vi "Process.vi"(8 "error in":errorcluster, 11 "Instrument.Lockin":refnum<class "Instrument.Lockin.lvclass">) -> (0 "error out":errorcluster, 3 "Instrument.Lockin out":refnum<class "Instrument.Lockin.lvclass">)   [LabVIEW 2019, in "Instrument.Lockin.lvlib" / "Instrument.Lockin.lvclass"]
doc: "---------------------------------------------------------------\nJKI State Machine Objects™\nhttp://jki.net/state-machine-objects/\nCopyright (C) 2005-2015, JKI <info@jki.net>\nALL RIGHTS RESERVED"
uses:
  Instrument.Lockin.lvclass
  C:/Program Files/National Instruments/LabVIEW 2019/vi.lib/JKI/JKI SMO/SMO/SMO.lvclass
  C:/Program Files/National Instruments/LabVIEW 2019/user.lib/LevyLab/Instrument Framework/Instrument/Instrument.lvclass
  Typedefs/API/Lockin.Commands.Local--Enum.ctl
  Instrument.Lockin.lvclass/Instrument.Lockin.ctl
  Typedefs/Lockin.Logging Mode--Enum.ctl
  Instrument.DAQ/Typedefs/PublicEvents--DAQ.getSweepWaveforms.ctl
  <vilib>/JKI/JKI SMO/SMO/SMO.lvclass/SMO.ctl
  Instrument.DAQ/Typedefs/Get State-enum.ctl
  26abb908-d0dd-4bb2-b0ae-9417a76ac08a.vi
  58bdca10-aee7-4643-9696-ab134e43fedf.vi
  57cf7fb7-944b-4fe2-b1a2-0684563889c1.vi
  f640c324-6c77-497d-a9f4-fdf294fa3808.vi
  2ccda5d8-d2df-4877-8897-cb36dbf858a1.vi
  7ebf71aa-15a6-4da8-8ab8-2681a3011f9e.vi
  befd05cc-8908-477d-a2f5-b8fbe5183ab0.vi
  4dcf9d6e-caf6-43ae-ab2a-813b64901b82.vi
  0479806f-3f82-4f4d-965e-31251a6a8c57.vi
  26abb908-d0dd-4bb2-b0ae-9417a76ac08a.vi/90a97669-4453-472b-bdf1-7bcd8eb08246.vi
  26abb908-d0dd-4bb2-b0ae-9417a76ac08a.vi/b26fcf18-2a8e-4202-9f3a-794c759f590f.vi
  58bdca10-aee7-4643-9696-ab134e43fedf.vi/a5cadab5-4a81-4843-8cd1-df529f160719.vi
  58bdca10-aee7-4643-9696-ab134e43fedf.vi/d6a5cc56-11f2-457d-8496-f6582433bdb5.vi
  57cf7fb7-944b-4fe2-b1a2-0684563889c1.vi/c78e9024-35b9-404a-847a-34b4f0e1b7cd.vi
  57cf7fb7-944b-4fe2-b1a2-0684563889c1.vi/9cccbff1-3b31-4ba5-974e-4119a5b66697.vi
  f640c324-6c77-497d-a9f4-fdf294fa3808.vi/fd9c0a75-bb1c-4df5-b428-97473e186f85.vi
  f640c324-6c77-497d-a9f4-fdf294fa3808.vi/5a332ac2-f3ee-43b7-a900-88e315d2e26c.vi
  2ccda5d8-d2df-4877-8897-cb36dbf858a1.vi/5836e187-7c61-41ed-8ee9-21d612ef42f8.vi
  2ccda5d8-d2df-4877-8897-cb36dbf858a1.vi/e16ae26d-577b-44d4-8830-38d114a60ef0.vi
  7ebf71aa-15a6-4da8-8ab8-2681a3011f9e.vi/4fe2dc9d-9353-45a3-b3dd-066009c5f601.vi
  7ebf71aa-15a6-4da8-8ab8-2681a3011f9e.vi/a83d1b05-35e4-4348-922d-f6ae74c7e255.vi
  befd05cc-8908-477d-a2f5-b8fbe5183ab0.vi/289e6158-3360-40af-af80-2e4dcd9b67a9.vi
  befd05cc-8908-477d-a2f5-b8fbe5183ab0.vi/5139ce6f-e826-4046-ae95-8880b2f2c8e2.vi
  4dcf9d6e-caf6-43ae-ab2a-813b64901b82.vi/c32a3efa-f786-486f-88c4-db6f71449899.vi
  4dcf9d6e-caf6-43ae-ab2a-813b64901b82.vi/a7bed843-5626-489a-9ac6-3c2874ac1268.vi
  0479806f-3f82-4f4d-965e-31251a6a8c57.vi/c63cbaba-d6ce-4e6f-84ba-6c88dbec8892.vi
  0479806f-3f82-4f4d-965e-31251a6a8c57.vi/12d99530-24f6-4df4-a18b-ab3b3e1e63e9.vi
  <vilib>/JKI/JKI SMO/SMO/Private/ReftoDVR--SMO.vi
  <vilib>/Utility/Data Type/Get Type Information.vi
  <vilib>/Utility/Data Type/Get Numeric Information.vi
  <userlib>/_OpenG.lib/lvdata/lvdata.llb/Unwrap VVariant__ogtk.vi
  <vilib>/JDP Science/JSONtext/Variant to JSON Text.vi
  <userlib>/LevyLab/Instrument Framework/Instrument/API/Instrument.sendMessageToProcess (string).vi
  <vilib>/JDP Science/JSONtext/LVClass Serializer/JSONtext LVClass Serializer.lvclass
  <userlib>/LevyLab/Instrument Framework/Instrument Types/Lockin/Instrument.LockinAPI.lvclass
  <userlib>/LevyLab/Debug/Debug.lvlib
  <userlib>/LevyLab/Instrument Framework/Instrument/Instrument.lvclass
  Instrument.DAQ/Instrument.DAQ.lvclass
  <vilib>/JKI/JKI SMO/SMO/SMO.lvclass
panel:
  in  "LOG":bool
  out "String":string
  # "Multichannel Lockin"
  # "For instructions on how to use the JKI State Machine Objects, examples and video tutorials, visit:\nhttp://jki.net/state-machine-objects/\n\nJKI State Machine Objects™\nhttp://jki.net/state-machine-objects/\nCopyright (C) 2005-2015, JKI <info@jki.net>\nALL RIGHTS RESERVED"
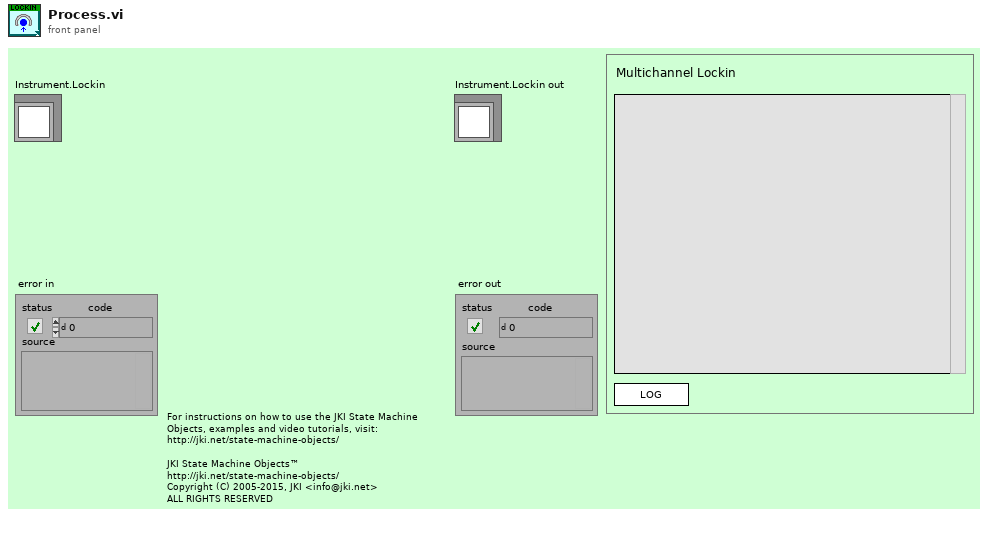
[diagram p1: front panel]
types:
  T1 = typedef "Instrument.Lockin.lvlib/Instrument.Lockin.lvclass/Lockin.Commands.Local--Enum.ctl" = enum16{"autoConfigureDAQ", "setSimulationMode", "zeroPhase", "setCalibration", "setPreFilter", "setLinkFrequencies", "setLimitAmplitude", "setLimitDC", "setSamplingDecimationPreDSP", "setSamplingDecimationPostDSP", "setSamplingMode", "setSamplingFsMultiplier", "setSamplingFsOutput", "setSamplingRefreshRate", "setData_State", "setData_DAQ", "setData_Sampling", "setData_Waveforms", "setData_Results", "setData_SweepWaveforms", "setData_AIChannels", "setData_AOChannels", "setData_REFChannels", "setData_InputGain", "setData_OutputGain", "showUI", "setAI", "setOffset", "setOffsetMode"}
  T2 = typedef "Instrument.Lockin.lvlib/Instrument.Lockin.lvclass/Lockin.Logging Mode--Enum.ctl" = enum16{"enabled", "disabled"}
  T3 = enum32{"invalid app kind", "Development System", "Run Time System", "Student Edition", "Embedded LabVIEW", "Evaluation", "Custom"}
  T4 = enum32{"Invalid", "Standard", "Closed", "Hidden", "Minimized", "Maximized"}
  T5 = typedef "Instrument.Lockin.lvlib/Instrument.DAQ.lvclass/Get State-enum.ctl" = enum16{"idle", "created", "started", "stopped", "sweeping"}
  T6 = typedef "Instrument.Lockin.lvlib/Instrument.DAQ.lvclass/PublicEvents--DAQ.getSweepWaveforms.ctl" = cluster{"AO_wfm":waveform(dbl)[], "AI_wfm":waveform(dbl)[], "X_wfm":waveform(dbl)[], "Y_wfm":waveform(dbl)[]}
  T7 = typedef "SMO.lvclass/SMOState --Enum.ctl" = enum16{"unknown", "Created", "Started", "Stopped"}
  T8 = cluster{"Core":cluster{"Current VI Reference":refnum<vi>, "Close Panel on Exit?":bool, "Last Error":cluster{"error":errorcluster, "previous state":string, "remaining states":string}, "Shutdown?":bool}, "SelfRef":refnum<class "Instrument.Lockin.lvclass">, "SweepWaveformsBuffer":T6}
  T9 = typedef "Instrument.Lockin.lvlib/Instrument.DAQ.lvclass/DAQ.Configuration--Cluster--Array.ctl" = T10[]
  T10 = typedef "Instrument.Lockin.lvlib/Instrument.DAQ.lvclass/DAQ.Configuration--Cluster.ctl" = cluster{"Device":string, "AO.Ch":string, "AO.Range":T11, "AI.Ch":string, "AI.Range":T12, "AI.Coupling":T13}
  T11 = typedef "Instrument.Lockin.lvlib/Instrument.DAQ.lvclass/DAQ.Config.AO.Range--enum.ctl" = enum16{"±0.1", "±1.0", "±10.0"}
  T12 = typedef "Instrument.Lockin.lvlib/Instrument.DAQ.lvclass/DAQ.Config.AI.Range--enum.ctl" = enum16{"±0.316", "±1.00", "±3.16", "±10.0", "±31.6", "±42.4"}
  T13 = typedef "Instrument.Lockin.lvlib/Instrument.DAQ.lvclass/DAQ.Config.AI.Coupling--enum.ctl" = u16
  T14 = typedef "Instrument.Lockin.lvlib/Instrument.DAQ.lvclass/DAQ.Config.AO--Cluster--Array.ctl" = T15[]
  T15 = typedef "Instrument.Lockin.lvlib/Instrument.DAQ.lvclass/DAQ.Config.AO--Cluster.ctl" = cluster{"Channels":tag, "Range":T11, "output terminal configuration":i32, "Type":T16}
  T16 = typedef "Instrument.Lockin.lvlib/Instrument.DAQ.lvclass/DAQ.Type--enum.ctl" = enum16{"None", "USB-4431", "PXI-446x"}
  T17 = typedef "Instrument.Lockin.lvlib/Instrument.DAQ.lvclass/DAQ.Config.AI--Cluster--Array.ctl" = T18[]
  T18 = typedef "Instrument.Lockin.lvlib/Instrument.DAQ.lvclass/DAQ.Config.AI--Cluster.ctl" = cluster{"Channels":tag, "Coupling":T13, "Range":T12, "input terminal configuration":i32, "Type":T16}
  T19 = typedef "Instrument.Lockin.lvlib/Instrument.DAQ.lvclass/DAQ.Sampling--Cluster.ctl" = cluster{"Sampling":T20, "sample mode":i32, "Fs Mode":T21, "Fs Multiplier":dbl, "Refresh Rate (Hz)":dbl, "Decimation.PreDSP":i32, "Decimation.PostDSP":i32, "Fs.Output":dbl}
  T20 = typedef "Instrument.Lockin.lvlib/Instrument.DAQ.lvclass/DAQ.Sampling.Sampling--Cluster.ctl" = cluster{"Fs":dbl, "#s":i32}
  T21 = typedef "Instrument.Lockin.lvlib/Instrument.DAQ.lvclass/DAQ.Sampling.Fs Mode--enum.ctl" = enum16{"Manual", "Auto Fs", "Max Fs"}
  T22 = typedef "Instrument.Lockin.lvlib/Instrument.DAQ.lvclass/AI.Channel--Cluster--Array.ctl" = T23[]
  T23 = typedef "Instrument.Lockin.lvlib/Instrument.DAQ.lvclass/AI.Channel--Cluster.ctl" = cluster{"Enable?":bool, "Channel":i32, "References":i32[]}
  T24 = typedef "Instrument.Lockin.lvlib/Instrument.DAQ.lvclass/AO.Channel--Cluster--Array.ctl" = T25[]
  T25 = typedef "Instrument.Lockin.lvlib/Instrument.DAQ.lvclass/AO.Channel--Cluster.ctl" = cluster{"Enable?":bool, "Channel":i32, "Amplitude":dbl, "Offset":dbl, "Frequency":dbl, "Phase":dbl, "Function":T26, "Sweeping?":bool}
  T26 = typedef "Instrument.Lockin.lvlib/Instrument.DAQ.lvclass/AO.Channel.Function--Enum.ctl" = enum16{"Sine", "Triangle", "Square"}
  T27 = typedef "Instrument.Lockin.lvlib/Instrument.DAQ.lvclass/REF.Channel--Cluster--Array.ctl" = T28[]
  T28 = typedef "Instrument.Lockin.lvlib/Instrument.DAQ.lvclass/REF.Channel--Cluster.ctl" = cluster{"Enable?":bool, "Channel":i32, "Frequency":dbl, "Phase":dbl, "TC":dbl, "Roll-Off":i32}
  T29 = typedef "Instrument.Lockin.lvlib/Instrument.DAQ.lvclass/PublicEvents--DAQ.getWaveforms.ctl" = cluster{"AO_wfm":waveform(dbl)[], "AI_wfm":waveform(dbl)[], "Ref_X_wfm":waveform(dbl)[], "Ref_Y_wfm":waveform(dbl)[], "X_wfm":waveform(dbl)[], "Y_wfm":waveform(dbl)[]}
  T30 = typedef "Instrument.Lockin.lvlib/Instrument.DAQ.lvclass/Results--Cluster.ctl" = cluster{"Time Stamp":timestamp, "Results (Dictionary)":cluster{"key":string, "value":dbl}[]}
  T31 = typedef "Instrument.Lockin.lvlib/Instrument.DAQ.lvclass/DeviceInfo--Cluster.ctl" = cluster{"DeviceName":string, "DevIsSimulated":bool, "DeviceSerialNumber":u32, "ProductType":string, "ProductCategory":i32, "ProductNumber":u32, "ChassisNumber":u32, "SlotNumber":u32, "ChassisName":string, "ChassisSerialNumber":u32}
  T32 = cluster{"Current VI Reference":refnum<vi>, "Close Panel on Exit?":bool, "Last Error":cluster{"error":errorcluster, "previous state":string, "remaining states":string}, "Shutdown?":bool}
  T33 = typedef "Debug.lvlib/Attribute.Debug.lvclass/DebugBehavior.ctl" = enum16{"Normal", "Debug"}
  T34 = typedef "SMO.lvclass/Protected Events.ctl" = cluster{"StopProcesses":refnum<user-event>, "AbortProcesses":refnum<user-event>, "Config Changed":refnum<user-event>, "Dependency":refnum<user-event>}
  T35 = typedef "SMO.lvclass/Public Events.ctl" = cluster{"Error":refnum<user-event>, "State":refnum<user-event>, "Reserve State":refnum<user-event>}
  T36 = typedef "Instrument.Lockin.lvlib/Instrument.DAQ.lvclass/PublicEvents--Cluster.ctl" = cluster{"getAIChannels":refnum<user-event>, "getAOChannels":refnum<user-event>, "getREFChannels":refnum<user-event>, "getWaveforms":refnum<user-event>, "getResults":refnum<user-event>, "getSweepWaveforms":refnum<user-event>, "getCalibration":refnum<user-event>, "getDAQState":refnum<user-event>, "getDAQconfig":refnum<user-event>, "getInputGain":refnum<user-event>, "getOutputGain":refnum<user-event>, "getInputOffset":refnum<user-event>, "getSampling":refnum<user-event>, "getSweepChannels":refnum<user-event>, "getDeviceIDN":refnum<user-event>}
  T37 = typedef "Instrument.Lockin.lvlib/Instrument.Lockin.lvclass/PrivateEvents--Cluster.ctl" = cluster{"Logging":refnum<user-event>}
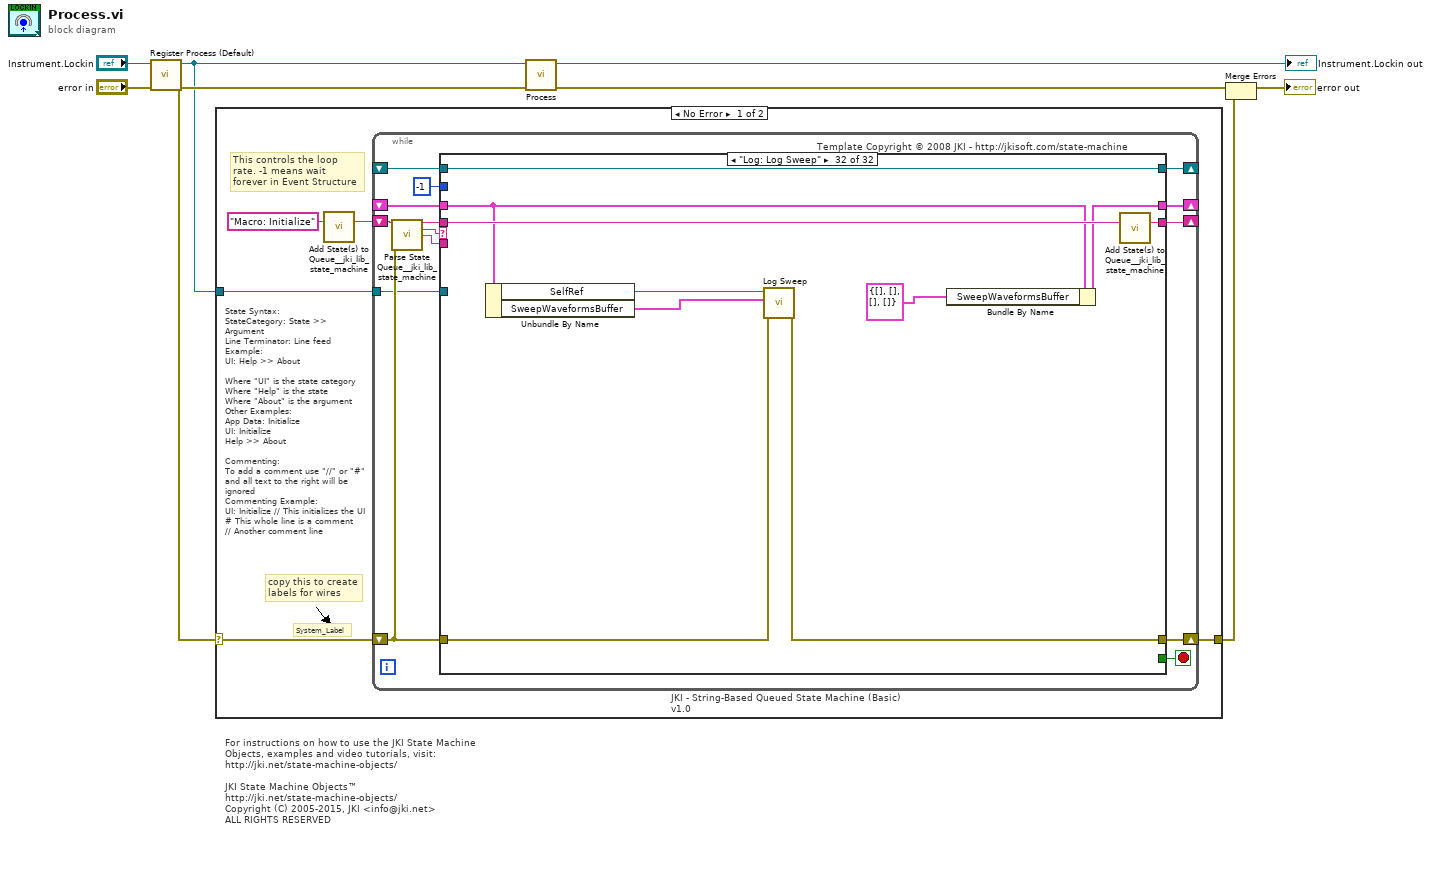
[diagram p0: block diagram]
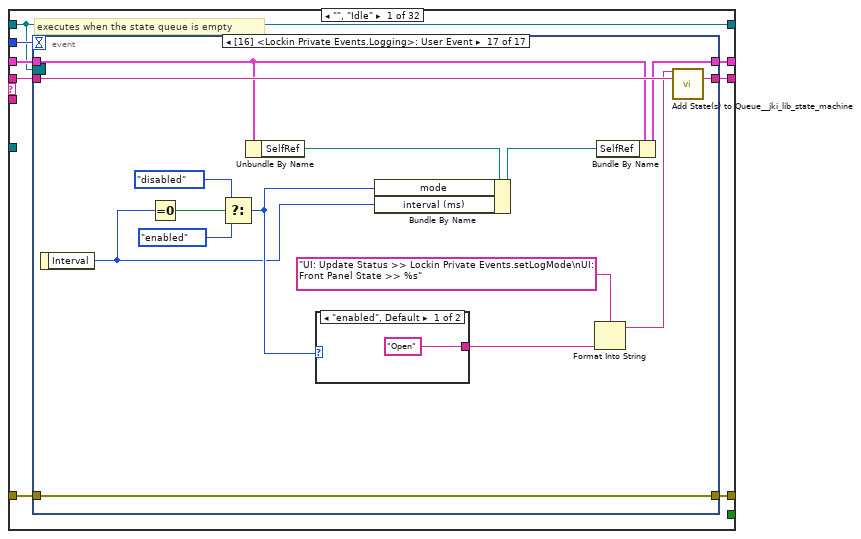
[diagram p2: hidden frame]
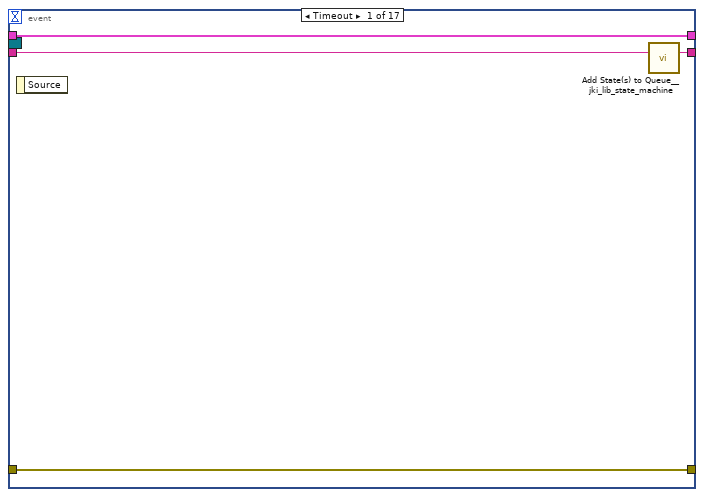
[diagram p3: hidden frame]
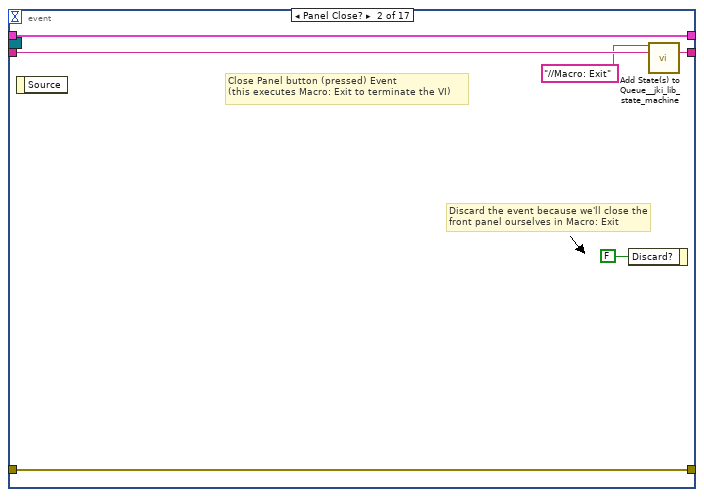
[diagram p4: hidden frame]
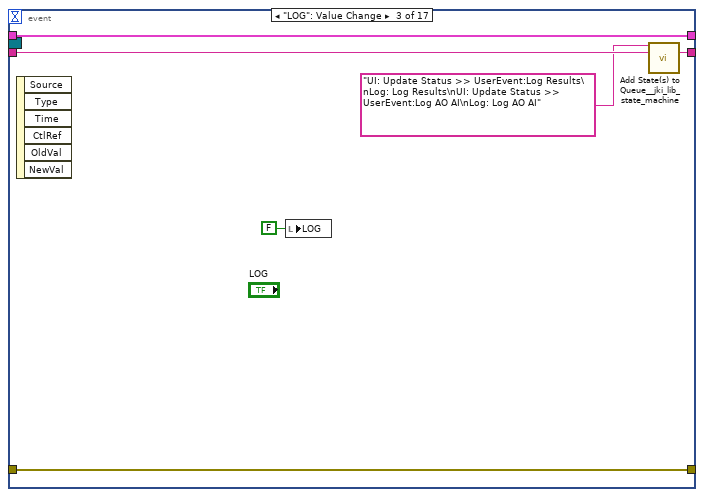
[diagram p5: hidden frame]
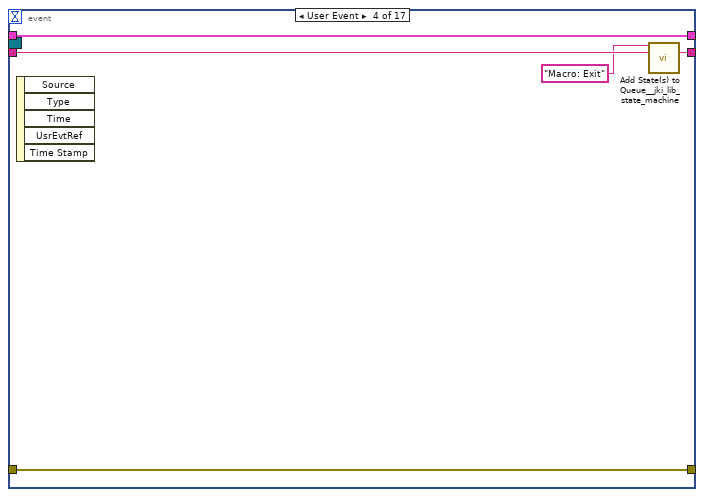
[diagram p6: hidden frame]
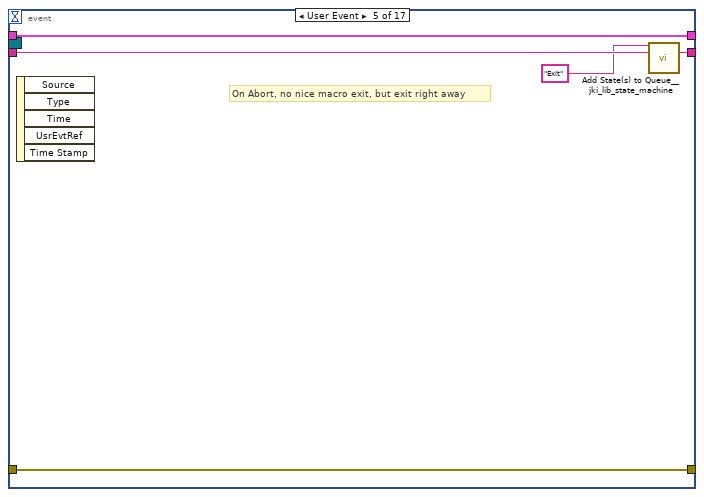
[diagram p7: hidden frame]
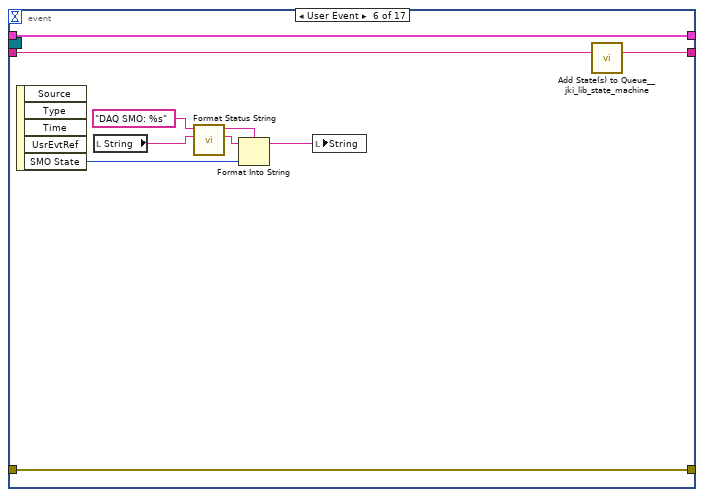
[diagram p8: hidden frame]
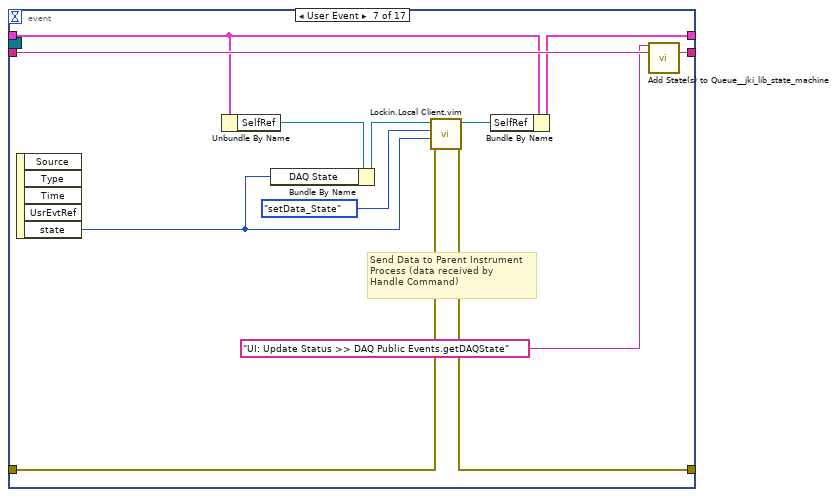
[diagram p9: hidden frame]
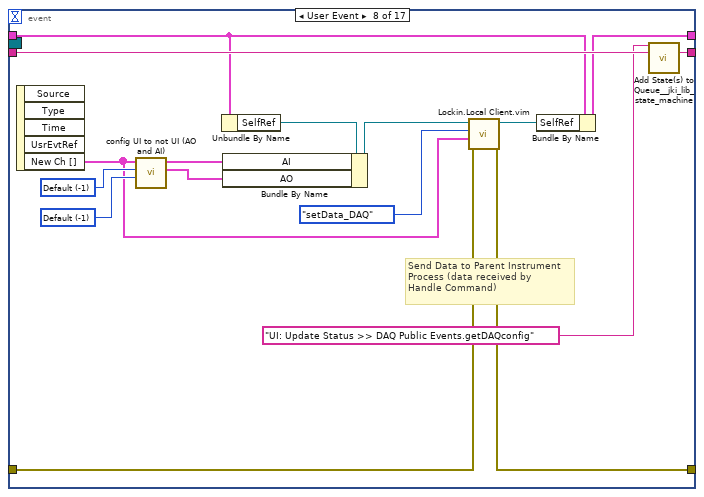
[diagram p10: hidden frame]
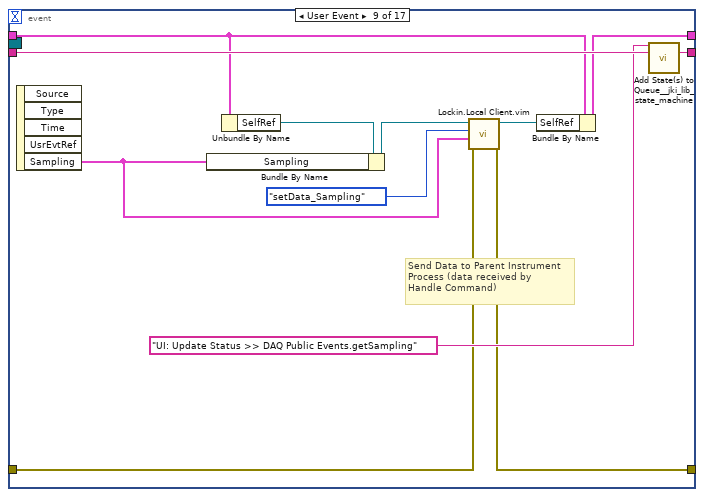
[diagram p11: hidden frame]
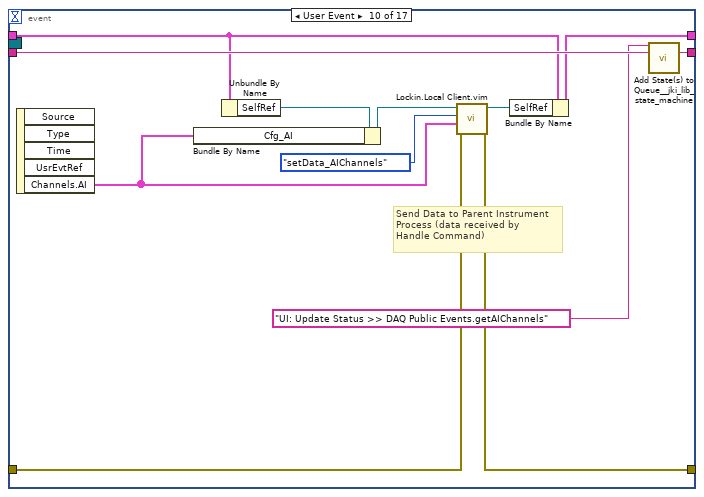
[diagram p12: hidden frame]
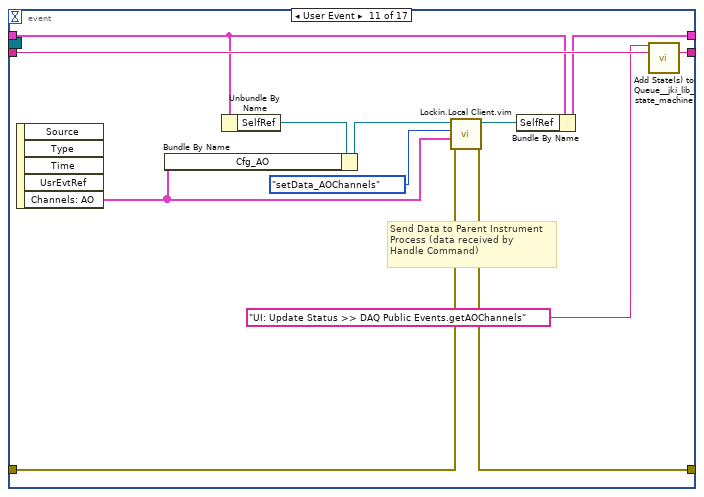
[diagram p13: hidden frame]
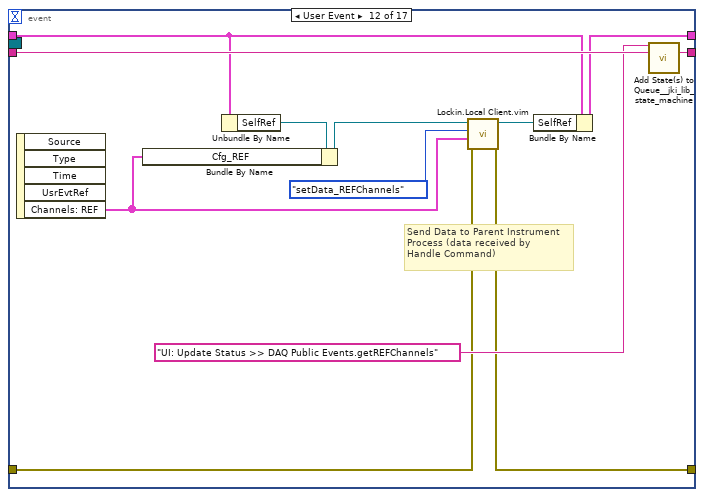
[diagram p14: hidden frame]
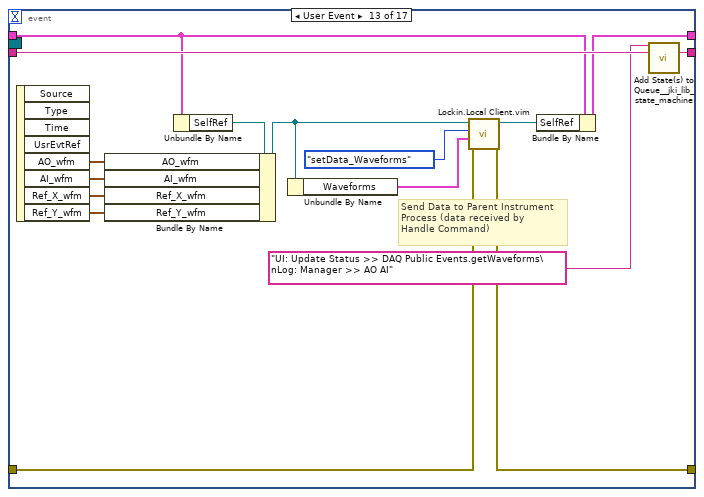
[diagram p15: hidden frame]
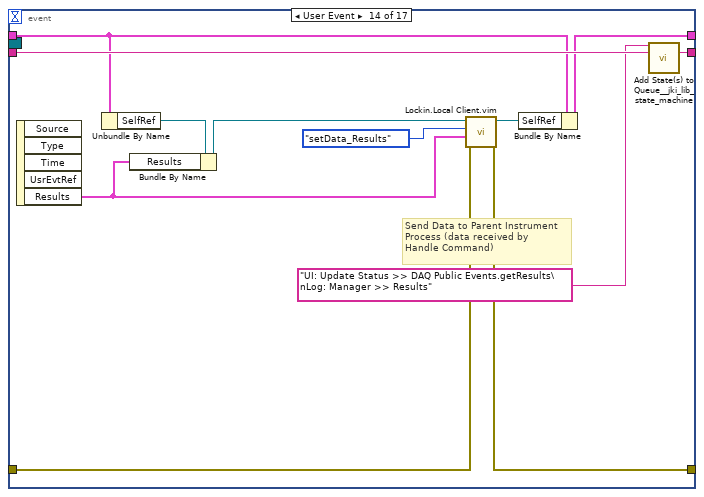
[diagram p16: hidden frame]
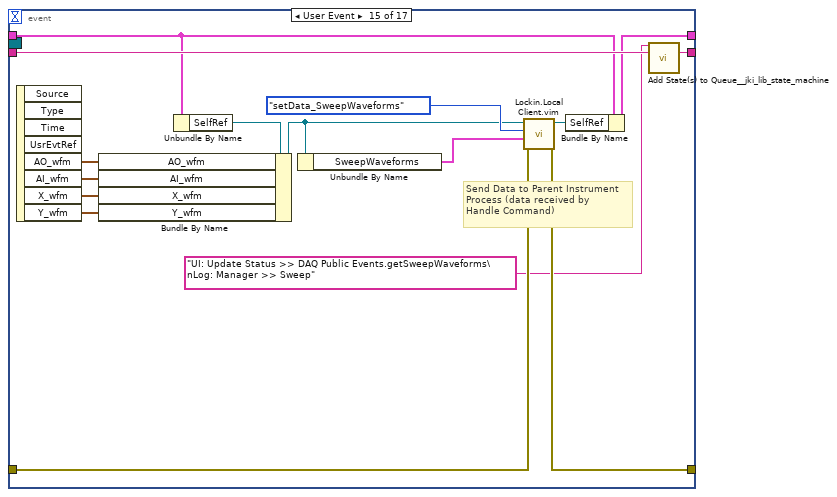
[diagram p17: hidden frame]
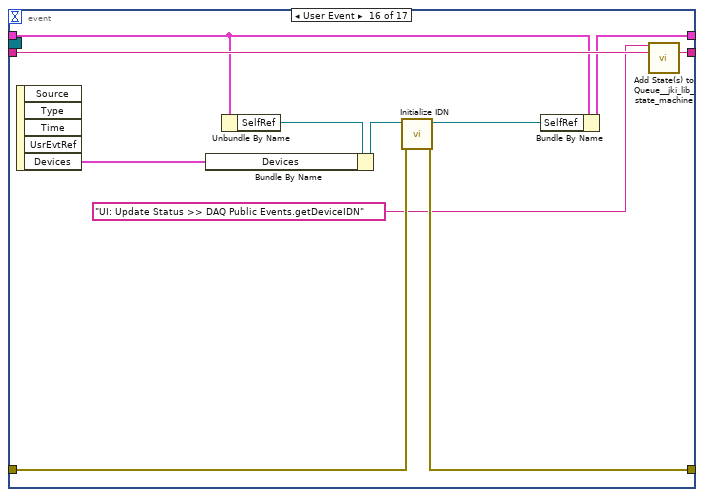
[diagram p18: hidden frame]
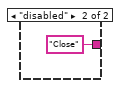
[diagram p19: hidden frame]
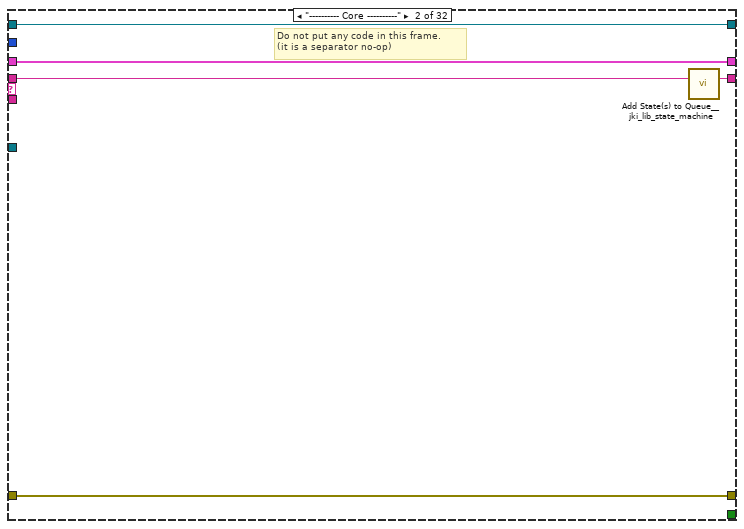
[diagram p20: hidden frame]
diagram:
  # "For instructions on how to use the JKI State Machine Objects, examples and video tutorials, visit:\nhttp://jki.net/state-machine-objects/\n\nJKI State Machine Objects™\nhttp://jki.net/state-machine-objects/\nCopyright (C) 2005-2015, JKI <info@jki.net>\nALL RIGHTS RESERVED"
  n1 = call <vilib>:"Register Process (Default).vi"("error in (no error)"="error in", "SMO"="Instrument.Lockin") -> ("error out"=w5:errorcluster, "SelfRef"=w4:refnum<class "Instrument.Lockin.lvclass">)  [unwired: 8 in]
  n2 = case shown="No Error" w5 {
    selector: w5 -> [w10 w574]
    tunnel: w4 -> [w11 _]
    tunnel: [w9 w574] -> w1
    frame No Error {
      # "State Syntax:\nStateCategory: State >> Argument\nLine Terminator: Line feed\nExample:\nUI: Help >> About\n\nWhere \"UI\" is the state category\nWhere \"Help\" is the state\nWhere \"About\" is the argument\nOther Examples:\nApp Data: Initialize\nUI: Initialize\nHelp >> About\n\nCommenting:\nTo add a comment use \"//\" or \"#\" and all text to the right will be ignored\nCommenting Example:\nUI: Initialize // This initializes the UI\n# This whole line is a comment\n// Another comment line"
      # "copy this to create labels for wires"
      # "This controls the loop rate. -1 means wait forever in Event Structure"
      # "System_Label"
      n3 = call <vilib>:"Add State(s) to Queue__jki_lib_state_machine.vi"("State(s) in (\"\")"="Macro: Initialize") -> ("States Out"=w13:string)  [unwired: 14 in]
      n4 = while "JKI - String-Based Queued State Machine (Basic) v1.0" {
        shift-right: [w20] -> _
        shift-left: _ -> [w19]
        shift-right: [w23] -> w9
        shift-left: w10 -> [w17]
        shift-right: [w22] -> _
        shift-left: w13 -> [w24]
        tunnel: w11 -> [w16]
        shift-right: [w15] -> _
        shift-left: _ -> [w14]
        stop <- w21 stop-if-true
        # "Template Copyright © 2008 JKI - http://jkisoft.com/state-machine"
        n5 = call <vilib>:"Parse State Queue__jki_lib_state_machine.vi"("State Queue"=w24, "Error In (no error)"=w17) -> ("Remaining States"=w26:string, "Current State"=w27:string, "Arguments"=w25:string)  [unwired: 11 in]
        n6 = case shown="\"Log: Log Sweep\"" w27 {
          selector: w27 -> [_ _ w226 _ _ _ _ _ _ _ _ _ _ _ _ _ _ _ _ _ _ _ _ _ _ _ _ _ _ _ _ _]
          tunnel: w26 -> [w35 w224 w230 w249 w251 w268 w273 w284 w291 w311 w316 w324 w331 w340 w347 w363 w395 w404 w416 w435 w456 w461 w472 w477 w494 w500 w505 w516 w549 w556 w563 w573]
          tunnel: w25 -> [_ _ _ _ _ _ _ _ _ _ _ _ w325 w332 w341 w357 _ _ _ _ _ _ _ _ _ _ _ w506 _ _ _ _]
          tunnel: w19 -> [w33 w221 w228 w240 w258 w264 w270 _ w286 w298 w313 w322 w328 w337 w345 w359 w392 w396 w405 w424 w441 w458 w469 w474 w488 w498 w501 w512 w546 w553 w560 w565]
          tunnel: [w32 w222 w232 w246 errorcluster {"status"=FALSE, "code"=0, "source"=""} ("No error") w263 w271 w280 w287 w309 w314 w319 w329 w338 w342 w360 w393 w398 w414 w422 w454 w459 w463 w475 w490 w496 w502 w513 w545 w552 w557 w568] -> w23
          tunnel: w17 -> [w31 w222 w231 w246 w260 _ w271 w280 w288 w309 w314 w318 w329 w338 w343 w361 w393 w398 w414 w421 w454 w459 w464 w475 w486 w496 w502 w513 w544 w550 w558 w569]
          tunnel: [w34 w223 w229 w248 w256 w267 w272 w283 w290 w310 w315 w323 w330 w339 w346 w362 w394 w403 w415 w434 w455 w460 w471 w476 w493 w499 w504 w515 w548 w555 w562 w572] -> w22
          tunnel: [_ _ _ _ _ TRUE _ _ _ _ _ _ _ _ _ _ _ _ _ _ _ _ _ _ _ _ _ _ _ _ _ _] -> w21
          tunnel: [w30 w221 w228 w247 w257 w264 w270 w282 w286 w299 w313 w322 w328 w337 w345 w359 w392 w396 w406 w425 w442 w458 w469 w474 w488 w498 w501 w512 w546 w553 w560 w566] -> w20
          tunnel: -1 ("Timeout") -> [w29 _ _ _ _ _ _ _ _ _ _ _ _ _ _ _ _ _ _ _ _ _ _ _ _ _ _ _ _ _ _ _]
          tunnel: w16 -> [_ _ _ _ _ _ _ w277 _ _ _ _ _ _ _ _ _ _ _ _ _ _ _ _ _ _ _ _ _ _ _ _]
          tunnel: [w28 w220 w225 w237 w262 w265 w269 w281 w285 w308 w312 w321 w327 w336 w344 w356 w391 w402 w413 w433 w448 w457 w470 w473 w492 w497 w503 w514 w547 w554 w561 w571] -> w15
          tunnel: w14 -> [w28 w220 w225 w237 w262 w265 w269 w281 w285 w308 w312 w321 w327 w336 w344 w356 w391 w402 w413 w433 w448 w457 w470 w473 _ w497 w503 w514 w547 w554 w561 w571]
          frame "", "Idle" {
            # "executes when the state queue is empty"
            n7 = event shown="[16] <Lockin Private Events.Logging>: User Event" {
              selector: w28 -> [_ _ _ _ _ _ _ _ _ _ _ _ _ _ _ _ _]
              dyn-events: _ -> [_ _ _ _ _ _ _ _ _ _ _ _ _ _ _ _ _]
              timeout: w29 -> [_ _ _ _ _ _ _ _ _ _ _ _ _ _ _ _ _]
              tunnel: w35 -> [w39 w45 w51 w56 w61 w69 w83 w99 w111 w123 w135 w147 w163 w175 w191 w202 w217]
              tunnel: [w38 w44 w50 w55 w60 w70 w82 w98 w110 w122 w134 w146 w162 w174 w190 w201 w216] -> w34
              tunnel: w33 -> [w36 w42 w48 w53 w58 w68 w80 w96 w108 w120 w132 w144 w160 w172 w188 w199 w214]
              tunnel: [w37 w43 w49 w54 w59 w67 w76 w86 w102 w117 w126 w137 w151 w170 w180 w194 w212] -> w32
              tunnel: w31 -> [w37 w43 w49 w54 w59 w67 w75 w85 w101 w116 w125 w136 w150 w169 w179 w193 w212]
              tunnel: [w36 w42 w48 w53 w58 w68 w81 w97 w109 w121 w133 w145 w161 w173 w189 w200 w215] -> w30
              event Timeout {
                n8 = event-data() -> ()  [unwired: 1 in, 1 out]
                n9 = call <vilib>:"Add State(s) to Queue__jki_lib_state_machine.vi"("State(s) in (\"\")"=w39) -> ("States Out"=w38:string)  [unwired: 14 in]
              }
              event Panel Close? {
                # "Discard the event because we'll close the front panel ourselves in Macro: Exit"
                # "Close Panel button (pressed) Event\n(this executes Macro: Exit to terminate the VI)"
                n10 = event-data() -> ()  [unwired: 1 in, 1 out]
                n11 = event-data("Discard?"=FALSE) -> ()  [unwired: 1 in, 1 out]
                n12 = call <vilib>:"Add State(s) to Queue__jki_lib_state_machine.vi"("State(s) in Front (\"\")"="//Macro: Exit", "State(s) in (\"\")"=w45) -> ("States Out"=w44:string)  [unwired: 13 in]
              }
              event "LOG": Value Change {
                n13 = event-data() -> ()  [unwired: 1 in, 6 out]
                n14 = local write "LOG"(FALSE ("LOG")) -> ()
                n15 = call <vilib>:"Add State(s) to Queue__jki_lib_state_machine.vi"("State(s) in Front (\"\")"="UI: Update Status >> UserEvent:Log Results\nLog: Log Results\nUI: Update Status >> UserEvent:Log AO AI\nLog: Log AO AI", "State(s) in (\"\")"=w51) -> ("States Out"=w50:string)  [unwired: 13 in]
              }
              event User Event {
                n16 = event-data() -> ()  [unwired: 1 in, 5 out]
                n17 = call <vilib>:"Add State(s) to Queue__jki_lib_state_machine.vi"("State(s) in Front (\"\")"="Macro: Exit", "State(s) in (\"\")"=w56) -> ("States Out"=w55:string)  [unwired: 13 in]
              }
              event User Event {
                # "On Abort, no nice macro exit, but exit right away"
                n18 = event-data() -> ()  [unwired: 1 in, 5 out]
                n19 = call <vilib>:"Add State(s) to Queue__jki_lib_state_machine.vi"("State(s) in Front (\"\")"="Exit", "State(s) in (\"\")"=w61) -> ("States Out"=w60:string)  [unwired: 13 in]
              }
              event User Event {
                n20 = event-data() -> ("SMO State"=w71:T7)  [unwired: 1 in, 4 out]
                n21 = local read "String"() -> (w64:string)
                n22 = call "Format Status String.vi"("initial string"=w64, "format string"="DAQ SMO: %s") -> ("initial string out"=w63:string, "format string out"=w62:string)  [unwired: 8 in]
                n23 = Format Into String(format string=w62, initial string=w63, w71) -> (resulting string=w66:string)  [unwired: 1 in, 1 out]
                n24 = local write "String"(w66) -> ()
                n25 = call <vilib>:"Add State(s) to Queue__jki_lib_state_machine.vi"("State(s) in (\"\")"=w69) -> ("States Out"=w70:string)  [unwired: 14 in]
              }
              event User Event {
                # "Send Data to Parent Instrument\nProcess (data received by\nHandle Command)"
                n26 = event-data() -> ("state"=w74:T5)  [unwired: 1 in, 4 out]
                n27 = Unbundle By Name(w80) -> ("SelfRef"=w73:refnum<class "Instrument.Lockin.lvclass">)
                n28 = Bundle By Name(cluster=w73, "DAQ State"=w74) -> (w72:refnum<class "Instrument.Lockin.lvclass">)
                n29 = call "Lockin.Local Client.vim"("error in (no error)"=w75, "Data"=w74, "Command"=Lockin.Commands.Local--Enum."setData_State" ("Enum"), "Instrument.Lockin in"=w72) -> ("error out"=w76:errorcluster, "Instrument.Lockin out"=w77:refnum<class "Instrument.Lockin.lvclass">)  [unwired: 6 in]
                n30 = Bundle By Name(cluster=w80, "SelfRef"=w77) -> (w81:T8)
                n31 = call <vilib>:"Add State(s) to Queue__jki_lib_state_machine.vi"("State(s) in Front (\"\")"="UI: Update Status >> DAQ Public Events.getDAQState" ("State(s) in Front (\"\")"), "State(s) in (\"\")"=w83) -> ("States Out"=w82:string)  [unwired: 13 in]
              }
              event User Event {
                w92 = -1 items=["Default"=-1, "RSE"=10083, "Differential"=10106, "Pseudodifferential"=12529] ("output terminal configuration")
                w93 = -1 items=["Default"=-1, "RSE"=10083, "NRSE"=10078, "Differential"=10106, "Pseudodifferential"=12529] ("input terminal configuration")
                # "Send Data to Parent Instrument\nProcess (data received by\nHandle Command)"
                n32 = event-data() -> ("New Ch []"=w87:T9)  [unwired: 1 in, 4 out]
                n33 = call "config UI to not UI (AO and AI).vi"("output terminal configuration"=w92, "input terminal configuration"=w93, "New Ch []"=w87) -> ("AO Config"=w90:T14, "AI Config"=w91:T17)  [unwired: 7 in]
                n34 = Unbundle By Name(w96) -> ("SelfRef"=w95:refnum<class "Instrument.Lockin.lvclass">)
                n35 = Bundle By Name(cluster=w95, "AI"=w91, "AO"=w90) -> (w89:refnum<class "Instrument.Lockin.lvclass">)
                n36 = call "Lockin.Local Client.vim"("error in (no error)"=w85, "Data"=w87, "Command"=Lockin.Commands.Local--Enum."setData_DAQ" ("Enum"), "Instrument.Lockin in"=w89) -> ("error out"=w86:errorcluster, "Instrument.Lockin out"=w88:refnum<class "Instrument.Lockin.lvclass">)  [unwired: 6 in]
                n37 = Bundle By Name(cluster=w96, "SelfRef"=w88) -> (w97:T8)
                n38 = call <vilib>:"Add State(s) to Queue__jki_lib_state_machine.vi"("State(s) in Front (\"\")"="UI: Update Status >> DAQ Public Events.getDAQconfig" ("State(s) in Front (\"\")"), "State(s) in (\"\")"=w99) -> ("States Out"=w98:string)  [unwired: 13 in]
              }
              event User Event {
                # "Send Data to Parent Instrument\nProcess (data received by\nHandle Command)"
                n39 = event-data() -> ("Sampling"=w100:T19)  [unwired: 1 in, 4 out]
                n40 = Unbundle By Name(w108) -> ("SelfRef"=w107:refnum<class "Instrument.Lockin.lvclass">)
                n41 = Bundle By Name(cluster=w107, "Sampling"=w100) -> (w104:refnum<class "Instrument.Lockin.lvclass">)
                n42 = call "Lockin.Local Client.vim"("error in (no error)"=w101, "Data"=w100, "Command"=Lockin.Commands.Local--Enum."setData_Sampling" ("Enum"), "Instrument.Lockin in"=w104) -> ("error out"=w102:errorcluster, "Instrument.Lockin out"=w103:refnum<class "Instrument.Lockin.lvclass">)  [unwired: 6 in]
                n43 = Bundle By Name(cluster=w108, "SelfRef"=w103) -> (w109:T8)
                n44 = call <vilib>:"Add State(s) to Queue__jki_lib_state_machine.vi"("State(s) in Front (\"\")"="UI: Update Status >> DAQ Public Events.getSampling" ("State(s) in Front (\"\")"), "State(s) in (\"\")"=w111) -> ("States Out"=w110:string)  [unwired: 13 in]
              }
              event User Event {
                # "Send Data to Parent Instrument\nProcess (data received by\nHandle Command)"
                n45 = event-data() -> ("Channels.AI"=w112:T22)  [unwired: 1 in, 4 out]
                n46 = Unbundle By Name(w120) -> ("SelfRef"=w119:refnum<class "Instrument.Lockin.lvclass">)
                n47 = Bundle By Name(cluster=w119, "Cfg_AI"=w112) -> (w115:refnum<class "Instrument.Lockin.lvclass">)
                n48 = call "Lockin.Local Client.vim"("error in (no error)"=w116, "Data"=w112, "Command"=Lockin.Commands.Local--Enum."setData_AIChannels" ("Enum"), "Instrument.Lockin in"=w115) -> ("error out"=w117:errorcluster, "Instrument.Lockin out"=w114:refnum<class "Instrument.Lockin.lvclass">)  [unwired: 6 in]
                n49 = Bundle By Name(cluster=w120, "SelfRef"=w114) -> (w121:T8)
                n50 = call <vilib>:"Add State(s) to Queue__jki_lib_state_machine.vi"("State(s) in Front (\"\")"="UI: Update Status >> DAQ Public Events.getAIChannels" ("State(s) in Front (\"\")"), "State(s) in (\"\")"=w123) -> ("States Out"=w122:string)  [unwired: 13 in]
              }
              event User Event {
                # "Send Data to Parent Instrument\nProcess (data received by\nHandle Command)"
                n51 = event-data() -> ("Channels: AO"=w128:T24)  [unwired: 1 in, 4 out]
                n52 = Unbundle By Name(w132) -> ("SelfRef"=w131:refnum<class "Instrument.Lockin.lvclass">)
                n53 = Bundle By Name(cluster=w131, "Cfg_AO"=w128) -> (w127:refnum<class "Instrument.Lockin.lvclass">)
                n54 = call "Lockin.Local Client.vim"("error in (no error)"=w125, "Data"=w128, "Command"=Lockin.Commands.Local--Enum."setData_AOChannels" ("Enum"), "Instrument.Lockin in"=w127) -> ("error out"=w126:errorcluster, "Instrument.Lockin out"=w124:refnum<class "Instrument.Lockin.lvclass">)  [unwired: 6 in]
                n55 = Bundle By Name(cluster=w132, "SelfRef"=w124) -> (w133:T8)
                n56 = call <vilib>:"Add State(s) to Queue__jki_lib_state_machine.vi"("State(s) in Front (\"\")"="UI: Update Status >> DAQ Public Events.getAOChannels" ("State(s) in Front (\"\")"), "State(s) in (\"\")"=w135) -> ("States Out"=w134:string)  [unwired: 13 in]
              }
              event User Event {
                # "Send Data to Parent Instrument\nProcess (data received by\nHandle Command)"
                n57 = event-data() -> ("Channels: REF"=w140:T27)  [unwired: 1 in, 4 out]
                n58 = Unbundle By Name(w144) -> ("SelfRef"=w143:refnum<class "Instrument.Lockin.lvclass">)
                n59 = Bundle By Name(cluster=w143, "Cfg_REF"=w140) -> (w139:refnum<class "Instrument.Lockin.lvclass">)
                n60 = call "Lockin.Local Client.vim"("error in (no error)"=w136, "Data"=w140, "Command"=Lockin.Commands.Local--Enum."setData_REFChannels" ("Enum"), "Instrument.Lockin in"=w139) -> ("error out"=w137:errorcluster, "Instrument.Lockin out"=w138:refnum<class "Instrument.Lockin.lvclass">)  [unwired: 6 in]
                n61 = Bundle By Name(cluster=w144, "SelfRef"=w138) -> (w145:T8)
                n62 = call <vilib>:"Add State(s) to Queue__jki_lib_state_machine.vi"("State(s) in Front (\"\")"="UI: Update Status >> DAQ Public Events.getREFChannels" ("State(s) in Front (\"\")"), "State(s) in (\"\")"=w147) -> ("States Out"=w146:string)  [unwired: 13 in]
              }
              event User Event {
                # "Send Data to Parent Instrument\nProcess (data received by\nHandle Command)"
                n63 = event-data() -> ("AO_wfm"=w158:waveform(dbl)[], "AI_wfm"=w157:waveform(dbl)[], "Ref_X_wfm"=w156:waveform(dbl)[], "Ref_Y_wfm"=w155:waveform(dbl)[])  [unwired: 1 in, 4 out]
                n64 = Unbundle By Name(w160) -> ("SelfRef"=w159:refnum<class "Instrument.Lockin.lvclass">)
                n65 = Bundle By Name(cluster=w159, "AO_wfm"=w158, "AI_wfm"=w157, "Ref_X_wfm"=w156, "Ref_Y_wfm"=w155) -> (w153:refnum<class "Instrument.Lockin.lvclass">)
                n66 = Unbundle By Name(w153) -> ("Waveforms"=w152:T29)
                n67 = call "Lockin.Local Client.vim"("error in (no error)"=w150, "Data"=w152, "Command"=Lockin.Commands.Local--Enum."setData_Waveforms" ("Enum"), "Instrument.Lockin in"=w153) -> ("error out"=w151:errorcluster, "Instrument.Lockin out"=w154:refnum<class "Instrument.Lockin.lvclass">)  [unwired: 6 in]
                n68 = Bundle By Name(cluster=w160, "SelfRef"=w154) -> (w161:T8)
                n69 = call <vilib>:"Add State(s) to Queue__jki_lib_state_machine.vi"("State(s) in Front (\"\")"="UI: Update Status >> DAQ Public Events.getWaveforms\nLog: Manager >> AO AI" ("State(s) in Front (\"\")"), "State(s) in (\"\")"=w163) -> ("States Out"=w162:string)  [unwired: 13 in]
              }
              event User Event {
                # "Send Data to Parent Instrument\nProcess (data received by\nHandle Command)"
                n70 = event-data() -> ("Results"=w167:T30)  [unwired: 1 in, 4 out]
                n71 = Unbundle By Name(w172) -> ("SelfRef"=w166:refnum<class "Instrument.Lockin.lvclass">)
                n72 = Bundle By Name(cluster=w166, "Results"=w167) -> (w165:refnum<class "Instrument.Lockin.lvclass">)
                n73 = call "Lockin.Local Client.vim"("error in (no error)"=w169, "Data"=w167, "Command"=Lockin.Commands.Local--Enum."setData_Results" ("Enum"), "Instrument.Lockin in"=w165) -> ("error out"=w170:errorcluster, "Instrument.Lockin out"=w168:refnum<class "Instrument.Lockin.lvclass">)  [unwired: 6 in]
                n74 = Bundle By Name(cluster=w172, "SelfRef"=w168) -> (w173:T8)
                n75 = call <vilib>:"Add State(s) to Queue__jki_lib_state_machine.vi"("State(s) in Front (\"\")"="UI: Update Status >> DAQ Public Events.getResults\nLog: Manager >> Results" ("State(s) in Front (\"\")"), "State(s) in (\"\")"=w175) -> ("States Out"=w174:string)  [unwired: 13 in]
              }
              event User Event {
                # "Send Data to Parent Instrument\nProcess (data received by\nHandle Command)"
                n76 = event-data() -> ("AO_wfm"=w186:waveform(dbl)[], "AI_wfm"=w185:waveform(dbl)[], "X_wfm"=w184:waveform(dbl)[], "Y_wfm"=w183:waveform(dbl)[])  [unwired: 1 in, 4 out]
                n77 = Unbundle By Name(w188) -> ("SelfRef"=w187:refnum<class "Instrument.Lockin.lvclass">)
                n78 = Bundle By Name(cluster=w187, "AO_wfm"=w186, "AI_wfm"=w185, "X_wfm"=w184, "Y_wfm"=w183) -> (w178:refnum<class "Instrument.Lockin.lvclass">)
                n79 = Unbundle By Name(w178) -> ("SweepWaveforms"=w177:T6)
                n80 = call "Lockin.Local Client.vim"("error in (no error)"=w179, "Data"=w177, "Command"=Lockin.Commands.Local--Enum."setData_SweepWaveforms" ("Enum"), "Instrument.Lockin in"=w178) -> ("error out"=w180:errorcluster, "Instrument.Lockin out"=w181:refnum<class "Instrument.Lockin.lvclass">)  [unwired: 6 in]
                n81 = Bundle By Name(cluster=w188, "SelfRef"=w181) -> (w189:T8)
                n82 = call <vilib>:"Add State(s) to Queue__jki_lib_state_machine.vi"("State(s) in Front (\"\")"="UI: Update Status >> DAQ Public Events.getSweepWaveforms\nLog: Manager >> Sweep" ("State(s) in Front (\"\")"), "State(s) in (\"\")"=w191) -> ("States Out"=w190:string)  [unwired: 13 in]
              }
              event User Event {
                n83 = event-data() -> ("Devices"=w198:T31[])  [unwired: 1 in, 4 out]
                n84 = Unbundle By Name(w199) -> ("SelfRef"=w197:refnum<class "Instrument.Lockin.lvclass">)
                n85 = Bundle By Name(cluster=w197, "Devices"=w198) -> (w196:refnum<class "Instrument.Lockin.lvclass">)
                n86 = call <userlib>:"Initialize IDN.vi"("error in (no error)"=w193, "Instrument in"=w196) -> ("error out"=w194:errorcluster, "Instrument out"=w195:refnum<class "Instrument.Lockin.lvclass">)  [unwired: 8 in]
                n87 = Bundle By Name(cluster=w199, "SelfRef"=w195) -> (w200:T8)
                n88 = call <vilib>:"Add State(s) to Queue__jki_lib_state_machine.vi"("State(s) in Front (\"\")"="UI: Update Status >> DAQ Public Events.getDeviceIDN" ("State(s) in Front (\"\")"), "State(s) in (\"\")"=w202) -> ("States Out"=w201:string)  [unwired: 13 in]
              }
              event User Event {
                n89 = event-data() -> ("Interval"=w203:u32)  [unwired: 1 in]
                n90 = Equal To 0?(x=w203) -> (x = 0?=w207:bool)
                n91 = Select(t=Lockin.Logging_Mode--Enum."disabled" ("Logging.Mode"), s=w207, f=Lockin.Logging_Mode--Enum."enabled" ("Logging.Mode")) -> (s? t:f=w204:T2)
                n92 = Unbundle By Name(w214) -> ("SelfRef"=w211:refnum<class "Instrument.Lockin.lvclass">)
                n93 = case shown="\"enabled\", Default" w204 {
                  tunnel: ["Open" ("input 1") "Close" ("input 1")] -> w208
                  frame "enabled", Default {
                  }
                  frame "disabled" {
                  }
                }
                n94 = Bundle By Name(cluster=w211, "mode"=w204, "interval (ms)"=w203) -> (w213:refnum<class "Instrument.Lockin.lvclass">)
                n95 = Format Into String(format string="UI: Update Status >> Lockin Private Events.setLogMode\nUI: Front Panel State >> %s" ("State(s) in Front (\"\")"), w208) -> (resulting string=w209:string)  [unwired: 2 in, 1 out]
                n96 = Bundle By Name(cluster=w214, "SelfRef"=w213) -> (w215:T8)
                n97 = call <vilib>:"Add State(s) to Queue__jki_lib_state_machine.vi"("State(s) in Front (\"\")"=w209, "State(s) in (\"\")"=w217) -> ("States Out"=w216:string)  [unwired: 13 in]
              }
            }
          }
          frame "---------- Core ----------" {
            # "Do not put any code in this frame.\n(it is a separator no-op)"
            n98 = call <vilib>:"Add State(s) to Queue__jki_lib_state_machine.vi"("State(s) in (\"\")"=w224) -> ("States Out"=w223:string)  [unwired: 14 in]
          }
          frame Default {
            w235 = 42 items=["No error", "Argument error", "Memory is full", "Out of zone", "End of file", "File already open", "Generic file I/O error", "File not found", "File permission error", "Disk is full", "Duplicate path", "Too many files open", "System feature not enabled", "Resource file not found", "Cannot add resource", "Resource not found", "Image not found", "Image memory error", "Pen does not exist", "Config type invalid", "Config token not found", "Config parse error", "Config memory error", "Bad external code format", "Bad external code offset", "External code not present", "Null window", "Destroy window error", "Null menu", "Print aborted", "Bad print record", "Print driver error", "Windows error during printing", "Memory error during printing", "Print dialog error", "Generic print error", "Invalid device refnum", "Device not found", "Device parameter error", "Device unit error", "Cannot open device", "Device call aborted", "Generic error", "Cancelled by user", "Object ID too low", "Object ID too high", "Object not in heap", "Unknown heap", "Unknown object (invalid DefProc)", "Unknown object (DefProc not in table)", "Message out of range", "Invalid (null) method", "Unknown message", "Manager call not supported", "Bad address", "Network operation in progress", "Network operation timed out", "Connection is busy", "Network attribute not supported", "Network error", "Address in use", "System out of memory", "Connection aborted", "Connection refused", "Not connected", "Already connected", "Connection closed", "Initialization error (interapplication manager)", "Bad occurrence", "Wait on unbound occurrence handler", "Occurrence queue overflow", "Datalog type conflict", "Unused", "Unrecognized type (interapplication manager)", "Memory corrupt", "Failed to make temporary DLL", "Old CIN version", "Drag socket not found", "Failed to load drop-object", "Failed to register OLE object", "Failed to release OLE object", "Format specifier type mismatch", "Unknown format specifier", "Too few format specifiers", "Too many format specifiers", "Scan failed", "Newer CIN version", "Error converting to variant", "Runtime menu error", "Password tampered", "Variant attribute not found", "Incompatible variant data type", "Event data is not available", "Event Store is not present", "Occurrence is not found", "Event Queue is not created", "Event info is not available", "Refnum passed is NULL", "Error retrieving Class GUID", "Error retrieving CoClass GUID", "Error retrieving TypeLib GUID.", "Bad built application magic bytes.", "Specific driver is different from the specific driver associated with the Logical Name.", "There is no session opened to the class driver.", "Max Error", "MAX - Error with config objects", "MAX - Error loading configuration", "MAX - Group not supported"]
            # "Current State"
            # "Do not delete, rename, or modify this frame.\n(this is used to capture unhandled states and typos)"
            # "Handle mistyped state name (developer tool)"
            n99 = Format Into String(format string="Software Exception: Unhandled State \"%s\"." ("message"), error in=w231, w226) -> (resulting string=w234:string, error out=w233:errorcluster)  [unwired: 1 in]
            n100 = call <vilib>:"Error Cluster From Error Code.vi"("show call chain? (False)"=TRUE, "error in (no error)"=w233, "error message (\"\")"=w234, "error code (0)"=w235) -> ("error out"=w232:errorcluster)  [unwired: 5 in]
            n101 = call <vilib>:"Add State(s) to Queue__jki_lib_state_machine.vi"("State(s) in (\"\")"=w230) -> ("States Out"=w229:string)  [unwired: 14 in]
          }
          frame "Initialize Core Data" {
            # "Do not delete, rename, or modify this frame.\n(this is used to determine panel behavior on exit)"
            # "originally closed?"
            # "exe?"
            # "If panel starts closed or is an EXE, then close it when we exit"
            n102 = property class="VI"() -> ("Front Panel.Open"=w245:bool)  [unwired: 2 in, 2 out]
            n103 = property class="App"() -> ("App.Kind"=w244:T3)  [unwired: 2 in, 2 out]
            n104 = control-ref of="Current VI Reference"() -> (w238:refnum<vi>)
            n105 = Not(x=w245) -> (.not. x?=w242:bool)
            n106 = Equal?(x=w244, y=T3."Run Time System" ("Application:Kind")) -> (x = y?=w241:bool)
            n107 = Or(x=w242, y=w241) -> (x .or. y?=w239:bool)
            n108 = Bundle By Name(cluster=w240, "Core.Current VI Reference"=w238, "Core.Close Panel on Exit?"=w239) -> (w247:T8)
            n109 = call <vilib>:"Add State(s) to Queue__jki_lib_state_machine.vi"("State(s) in (\"\")"=w249) -> ("States Out"=w248:string)  [unwired: 14 in]
          }
          frame "Error Handler" {
            w252 = FALSE  # Stop on Unhandled Error (T)
            # "Clear error"
            # "There was an error while handling the error.\nStop the process. This error can only occur if public events references are invalid or if the state machine object is destroyed."
            # "Overwrite this method to handle errors and pass to parent if not handled. Parent will fire a public event if the error is not handled up the chain of classes."
            n110 = Unbundle By Name(w258) -> ("SelfRef"=w261:refnum<class "Instrument.Lockin.lvclass">)
            n111 = call-dynamic "Handle Error.vi"("Stop on Unhandled Error (T)"=w252, "error in"=w260, "SMO"=w261) -> ("handling error"=w253:errorcluster, "Unhandled error"=w255:errorcluster)  [unwired: 6 in, 1 out]
            n112 = Bundle By Name(cluster=w258, "Core.Last Error.remaining states"=w251, "Core.Last Error.error"=w255) -> (w257:T8)
            n113 = Select(t="Exit", s=w253, f="Macro: Post Error Handling") -> (s? t:f=w256:string)
          }
          frame "Exit" {
            # "Do not put any code in this frame.\n(No errors that occur here will be handled.)"
            n114 = Unbundle By Name(w264) -> ("Core.Last Error.error"=w263:errorcluster)
            n115 = call <vilib>:"Add State(s) to Queue__jki_lib_state_machine.vi"("State(s) in (\"\")"=w268) -> ("States Out"=w267:string)  [unwired: 14 in]
          }
          frame "---------- Data ----------" {
            # "Do not put any code in this frame.\n(It is a separator no-op. You can make a copy of this frame to create a new Data frame)"
            n116 = call <vilib>:"Add State(s) to Queue__jki_lib_state_machine.vi"("State(s) in (\"\")"=w273) -> ("States Out"=w272:string)  [unwired: 14 in]
          }
          frame "Data: Initialize" {
            w276 = T6 {"AO_wfm"=[], "AI_wfm"=[], "X_wfm"=[], "Y_wfm"=[]}  # SweepWaveformsBuffer
            w279 = T32 {"Current VI Reference"=refnum, "Close Panel on Exit?"=FALSE, "Last Error"={"error"={"status"=FALSE, "code"=0, "source"=""}, "previous state"="", "remaining states"=""}, "Shutdown?"=FALSE}  # Core
            # "do not delete - used by framework"
            # "Data names and types of shift register data are defined by this bundle."
            # "Initialize the shift-register data, here.\n(data names are defined by what you wire into the bundle function)"
            n117 = Bundle By Name(cluster=w277, "mode"=Lockin.Logging_Mode--Enum."disabled" ("Mode"), "interval (ms)"=u32 1000 ("Logging.Interval (s)")) -> (w278:refnum<class "Instrument.Lockin.lvclass">)
            n118 = Bundle("Core"=w279, "SelfRef"=w278, "SweepWaveformsBuffer"=w276) -> (w282:T8)  [unwired: 1 in]
            n119 = call <vilib>:"Add State(s) to Queue__jki_lib_state_machine.vi"("State(s) in (\"\")"=w284) -> ("States Out"=w283:string)  [unwired: 14 in]
          }
          frame "Data: Cleanup" {
            # "Cleanup any data and references, here.\n(this is called automatically, by the Macro: Exit)"
            n120 = Unbundle By Name(w286) -> ("Core.Current VI Reference"=w289:refnum<vi>)
            n121 = Close Reference(reference=w289, error in (no error)=w288) -> (error out=w287:errorcluster)
            n122 = call <vilib>:"Add State(s) to Queue__jki_lib_state_machine.vi"("State(s) in (\"\")"=w291) -> ("States Out"=w290:string)  [unwired: 14 in]
          }
          frame "Data: Buffer" {
            # "Do not put any code in this frame.\n(It is a separator no-op. You can make a copy of this frame to create a new Data frame)"
            n123 = Unbundle By Name(w298) -> ("SweepWaveformsBuffer"=w301:T6, "SelfRef"=w307:refnum<class "Instrument.Lockin.lvclass">)
            n124 = Unbundle By Name(w307) -> ("AO_wfm"=w306:waveform(dbl)[], "AI_wfm"=w305:waveform(dbl)[], "X_wfm"=w304:waveform(dbl)[], "Y_wfm"=w302:waveform(dbl)[])
            n125 = Unbundle By Name(w301) -> ("AO_wfm"=w293:waveform(dbl)[], "AI_wfm"=w292:waveform(dbl)[], "X_wfm"=w295:waveform(dbl)[], "Y_wfm"=w303:waveform(dbl)[])
            n126 = call "Waveform Buffer.vi"("Waveform B []"=w304, "Waveforrm A []"=w295) -> ("Waveform out []"=w294:waveform(dbl)[])  [unwired: 8 in, 1 out]
            n127 = call "Waveform Buffer.vi"("Waveform B []"=w306, "Waveforrm A []"=w293) -> ("Waveform out []"=w297:waveform(dbl)[])  [unwired: 8 in, 1 out]
            n128 = call "Waveform Buffer.vi"("Waveform B []"=w305, "Waveforrm A []"=w292) -> ("Waveform out []"=w296:waveform(dbl)[])  [unwired: 8 in, 1 out]
            n129 = call "Waveform Buffer.vi"("Waveform B []"=w302, "Waveforrm A []"=w303) -> ("Waveform out []"=w300:waveform(dbl)[])  [unwired: 8 in, 1 out]
            n130 = Bundle By Name(cluster=w298, "SweepWaveformsBuffer.AO_wfm"=w297, "SweepWaveformsBuffer.AI_wfm"=w296, "SweepWaveformsBuffer.X_wfm"=w294, "SweepWaveformsBuffer.Y_wfm"=w300) -> (w299:T8)
            n131 = call <vilib>:"Add State(s) to Queue__jki_lib_state_machine.vi"("State(s) in (\"\")"=w311) -> ("States Out"=w310:string)  [unwired: 14 in]
          }
          frame "---------- UI ----------" {
            # "Do not put any code in this frame.\n(It is a separator no-op. You can make a copy of this frame to create a new UI frame)"
            n132 = call <vilib>:"Add State(s) to Queue__jki_lib_state_machine.vi"("State(s) in (\"\")"=w316) -> ("States Out"=w315:string)  [unwired: 14 in]
          }
          frame "UI: Initialize" {
            # "Initialize the User Interface, here.\n(this is called automatically, by the Macro: Init)"
            n133 = call <userlib>:"Fit VI window to Largest Dec__ogtk.vi"("error in (no error)"=w318, "border spacing (2 px)"=0) -> ("error out"=w319:errorcluster)  [unwired: 4 in, 1 out]
            n134 = call <vilib>:"Add State(s) to Queue__jki_lib_state_machine.vi"("State(s) in (\"\")"=w324) -> ("States Out"=w323:string)  [unwired: 14 in]
            "String" <- "" ("String")
          }
          frame "UI: Update Status" {
            n135 = call <userlib>:"State History.vi"("Current State"=w325) -> ("History"=w326:string)  [unwired: 10 in]
            n136 = local write "String"(w326) -> ()
            n137 = call <vilib>:"Add State(s) to Queue__jki_lib_state_machine.vi"("State(s) in (\"\")"=w331) -> ("States Out"=w330:string)  [unwired: 14 in]
          }
          frame "UI: Wait" {
            # "Do not put any code in this frame.\n(It is a separator no-op. You can make a copy of this frame to create a new UI frame)"
            n138 = Scan From String(format string="%d", input string=w332, default 1=u32 0 ("default value 1")) -> (output 1=w333:u32)  [unwired: 2 in, 3 out]
            n139 = Wait (ms)(milliseconds to wait=w333) -> ()  [unwired: 1 out]
            n140 = call <vilib>:"Add State(s) to Queue__jki_lib_state_machine.vi"("State(s) in (\"\")"=w340) -> ("States Out"=w339:string)  [unwired: 14 in]
          }
          frame "UI: Cursor Set" {
            # "Argument"
            # "Initialize the User Interface, here.\n(this is called automatically, by the Macro: Init)"
            n141 = disable-structure shown="Default" {
              disable-tunnel: w343 -> [w348 w351]
              disable-tunnel: [w348 w350] -> w342
              disable-tunnel: w341 -> [_ w349]
              frame condition #0 {
              }
              frame condition #1 (active) {
                n142 = case shown="\"Idle\", Default" w349 {
                  tunnel: w351 -> [w353 w355]
                  tunnel: [w352 w354] -> w350
                  frame "Idle", Default {
                    n143 = call <vilib>:"Unset Busy.vi"("error in (no error)"=w353) -> ("error out"=w352:errorcluster)  [unwired: 10 in]
                  }
                  frame "Busy" {
                    n144 = call <vilib>:"Set Busy.vi"("error in (no error)"=w355) -> ("error out"=w354:errorcluster)  [unwired: 9 in, 1 out]
                  }
                }
              }
            }
            n145 = call <vilib>:"Add State(s) to Queue__jki_lib_state_machine.vi"("State(s) in (\"\")"=w347) -> ("States Out"=w346:string)  [unwired: 14 in]
          }
          frame "UI: Front Panel State" {
            # "Argument"
            # "Set Front Panel Open or Closed\n(Usage: \"UI: Front Panel State >> Open|Close\")"
            n146 = Unbundle By Name(w359) -> ("Core.Current VI Reference"=w358:refnum<vi>)
            n147 = disable-structure shown="Default" {
              disable-tunnel: w361 -> [w367 w390]
              disable-tunnel: [w366 w390] -> w360
              disable-tunnel: w358 -> [w365 _]
              disable-tunnel: w357 -> [w364 _]
              frame condition #0 (active) {
                n148 = case shown="\"Close\"" w364 {
                  tunnel: w367 -> [w371 w384]
                  tunnel: [w373 w385] -> w366
                  tunnel: w365 -> [w372 w382]
                  frame "Open", Default {
                    n149 = property class="VI"(reference=w372, error in=w371) -> (reference out=w369:refnum<vi>, error out=w370:errorcluster, "FP.State"=w368:T4)
                    n150 = case shown="\"Closed\"" w368 {
                      tunnel: [w376 w379] -> w373
                      tunnel: w370 -> [w375 w379]
                      tunnel: w369 -> [w374 _]
                      frame "Closed" {
                        n151 = invoke class="VI" method="FP.Open"(reference=w374, error in=w375, "Activate"=TRUE, "State"=T4."Standard") -> (error out=w376:errorcluster)  [unwired: 1 in, 4 out]
                      }
                      frame Default {
                      }
                    }
                  }
                  frame "Close" {
                    n152 = property class="VI"(reference=w382, error in=w384) -> (reference out=w381:refnum<vi>, error out=w383:errorcluster, "FP.State"=w380:T4)
                    n153 = case shown="Default" w380 {
                      tunnel: [w386 w389] -> w385
                      tunnel: w383 -> [w386 w388]
                      tunnel: w381 -> [_ w387]
                      frame "Invalid", "Closed" {
                      }
                      frame Default {
                        n154 = invoke class="VI" method="FP.Close"(reference=w387, error in=w388) -> (error out=w389:errorcluster)  [unwired: 1 in, 2 out]
                      }
                    }
                  }
                }
              }
              frame condition #1 {
              }
            }
            n155 = call <vilib>:"Add State(s) to Queue__jki_lib_state_machine.vi"("State(s) in (\"\")"=w363) -> ("States Out"=w362:string)  [unwired: 14 in]
          }
          frame "---------- Macro ----------" {
            # "Do not put any code in this frame.\n(It is a separator no-op. You can make a copy of this frame to create a new Macro frame)"
            n156 = call <vilib>:"Add State(s) to Queue__jki_lib_state_machine.vi"("State(s) in (\"\")"=w395) -> ("States Out"=w394:string)  [unwired: 14 in]
          }
          frame "Macro: Initialize" {
            w397 = "UI: Initialize\nUI: Front Panel State >> Open\nMacro: Debug"  # UI: Initialize UI: Front Panel State >> Open Macro: Debug
            # "Initialization Macro\n(This is called once, when the VI starts)"
            n157 = call <vilib>:"Add State(s) to Queue__jki_lib_state_machine.vi"("State(s) in Front (\"\")"="Data: Initialize\nInitialize Core Data\nEvents: Register", "State(s) in (\"\")"="Process: Sync", "State(s) at Back (\"\")"=w397) -> ("States Out"=w400:string)  [unwired: 12 in]
            n158 = call <vilib>:"Add State(s) to Queue__jki_lib_state_machine.vi"("State(s) in Front (\"\")"=w400, "State(s) in (\"\")"=w404) -> ("States Out"=w403:string)  [unwired: 13 in]
          }
          frame "Macro: Post Error Handling" {
            # "Clear Last Error?"
            n159 = Unbundle By Name(w405) -> ("Core.Last Error.remaining states"=w408:string, "Core.Shutdown?"=w409:bool)
            n160 = Unbundle By Name(w405) -> ("Core.Last Error.error"=w412:errorcluster)
            n161 = case shown="False" FALSE {
              tunnel: w412 -> [w420 _]
              tunnel: [w420 _] -> w411
              frame False {
              }
              frame True {
              }
            }
            n162 = case shown="False" w409 {
              tunnel: w408 -> [w417 w419]
              tunnel: [w417 w418] -> w407
              frame False {
                # "These are the remaining states (at the moment the error occured). States can be altered according to business logic."
                # "NOT SHUTTING DOWN"
              }
              frame True {
                # "Developer can decide to alter the states but should be aware that during the shutdown process, there are certain states that must be run for the SMO to properly shut itself (and this process) down. As such, one can add states to perform additional clean-ups, but should append the remaining state to be executed."
                # "SHUTTING DOWN"
                n163 = call <vilib>:"Add State(s) to Queue__jki_lib_state_machine.vi"("State(s) in (\"\")"=w419) -> ("States Out"=w418:string)  [unwired: 14 in]
              }
            }
            n164 = Bundle By Name(cluster=w405, "Core.Last Error.error"=w411) -> (w406:T8)
            n165 = call <vilib>:"Add State(s) to Queue__jki_lib_state_machine.vi"("State(s) in Front (\"\")"=w407, "State(s) in (\"\")"=w416) -> ("States Out"=w415:string)  [unwired: 13 in]
          }
          frame "Macro: Debug" {
            # "exe?"
            # "If pane is an EXE, then close it when we exit"
            # "Macro: Debug\n(get debug behavior, determine UI and determine shutdown behavior)"
            n166 = Unbundle By Name(w424) -> ("Core.Close Panel on Exit?"=w427:bool, "SelfRef"=w432:refnum<class "Instrument.Lockin.lvclass">)
            n167 = property class="App"() -> ("App.Kind"=w430:T3)  [unwired: 2 in, 2 out]
            n168 = Equal?(x=w430, y=T3."Run Time System" ("Application:Kind")) -> (x = y?=w426:bool)
            n169 = call <userlib>:"Get Debug Mode.vi"("error in (no error)"=w421, "SMO"=w432) -> ("error out"=w422:errorcluster, "Behavior"=w431:T33)  [unwired: 7 in, 1 out]
            n170 = case shown="\"Normal\", Default" w431 {
              tunnel: [w436 w438] -> w428
              tunnel: w427 -> [w436 _]
              tunnel: w426 -> [_ w440]
              tunnel: [_ "UI: Front Panel State >> Open\nUI: Wait >> 1000"] -> w423
              frame "Normal", Default {
                # "respect core.close"
              }
              frame "Debug" {
                # "keep panel open\nunless exe"
                n171 = Or(x=w440, y=FALSE) -> (x .or. y?=w438:bool)
              }
            }
            n172 = Bundle By Name(cluster=w424, "Core.Close Panel on Exit?"=w428) -> (w425:T8)
            n173 = call <vilib>:"Add State(s) to Queue__jki_lib_state_machine.vi"("State(s) in Front (\"\")"=w423, "State(s) in (\"\")"=w435) -> ("States Out"=w434:string)  [unwired: 13 in]
          }
          frame "Macro: Exit" {
            # "Exit Macro\n(This is called once, when the VI exits)"
            n174 = Unbundle By Name(w441) -> ("Core.Close Panel on Exit?"=w453:bool)
            n175 = Bundle By Name(cluster=w441, "Core.Shutdown?"=TRUE) -> (w442:T8)
            n176 = Select(t="UI: Front Panel State >> Close", s=w453, f="") -> (s? t:f=w450:string)
            n177 = call <vilib>:"Add State(s) to Queue__jki_lib_state_machine.vi"("State(s) in Front (\"\")"="Data: Cleanup\nEvents: Unregister", "State(s) in (\"\")"="Process: Sync", "State(s) at Back (\"\")"="Exit") -> ("States Out"=w445:string)  [unwired: 12 in]
            n178 = call <vilib>:"Add State(s) to Queue__jki_lib_state_machine.vi"("State(s) in (\"\")"=w450, "State(s) at Back (\"\")"=w445) -> ("States Out"=w449:string)  [unwired: 13 in]
            n179 = call <vilib>:"Add State(s) to Queue__jki_lib_state_machine.vi"("State(s) in Front (\"\")"=w449, "State(s) in (\"\")"=w456) -> ("States Out"=w455:string)  [unwired: 13 in]
          }
          frame "---------- Process ----------" {
            # "Template Separator\n(You can make a copy of, or modify, this frame)"
            n180 = call <vilib>:"Add State(s) to Queue__jki_lib_state_machine.vi"("State(s) in (\"\")"=w461) -> ("States Out"=w460:string)  [unwired: 14 in]
          }
          frame "Process: Sync" {
            n181 = Unbundle By Name(w469) -> ("SelfRef"=w465:refnum<class "Instrument.Lockin.lvclass">)
            n182 = call <vilib>:"WaitOnProcessSync.vi"("error in (no error)"=w464, "SMO"=w465) -> ("error out"=w463:errorcluster, "Don't run?"=w468:bool)  [unwired: 7 in, 1 out]
            n183 = Select(t="Data: Cleanup\nEvents: Unregister\nExit", s=w468, f="") -> (s? t:f=w462:string)
            n184 = call <vilib>:"Add State(s) to Queue__jki_lib_state_machine.vi"("State(s) in Front (\"\")"=w462, "State(s) in (\"\")"=w472) -> ("States Out"=w471:string)  [unwired: 13 in]
          }
          frame "---------- Events ----------" {
            # "Template Separator\n(You can make a copy of, or modify, this frame)"
            n185 = call <vilib>:"Add State(s) to Queue__jki_lib_state_machine.vi"("State(s) in (\"\")"=w477) -> ("States Out"=w476:string)  [unwired: 14 in]
          }
          frame "Events: Register" {
            # "Expand to add\nmore events"
            n186 = Unbundle By Name(w488) -> ("SelfRef"=w487:refnum<class "Instrument.Lockin.lvclass">)
            n187 = call <vilib>:"GetProtectedEvents.vi"("SMO"=w487) -> ("error out"=w489:errorcluster, "SMO Protected Events"=w491:T34, "SMO out"=w482:refnum<class "Instrument.Lockin.lvclass">)  [unwired: 8 in]
            n188 = call "Lockin.getDAQPublicEvents.vi"("Instrument.Lockin in"=w482) -> ("error out"=w483:errorcluster, "DAQ SMO Public Events"=w481:T35, "DAQ Public Events"=w484:T36, "Instrument.Lockin out"=w480:refnum<class "Instrument.Lockin.lvclass">)  [unwired: 7 in]
            n189 = call "Lockin.GetPrivateEvents.vi"("Instrument.Lockin in"=w480) -> ("error out"=w478:errorcluster, "Lockin Private Events"=w479:T37)  [unwired: 8 in, 1 out]
            n190 = register-events(w491, w484, w481, w479) -> (reference out=w492:refnum<event-registration>, error out=w485:errorcluster)  [unwired: 2 in]
            n191 = Merge Errors(w485, w478, w483, w489, w486) -> (w490:errorcluster)
            n192 = call <vilib>:"Add State(s) to Queue__jki_lib_state_machine.vi"("State(s) in (\"\")"=w494) -> ("States Out"=w493:string)  [unwired: 14 in]
          }
          frame "Events: Unregister" {
            n193 = Unregister For Events(event registration refnum=w497, error in=w496) -> (error out=w495:errorcluster)
            n194 = call <vilib>:"Clear Errors.vi"("error in (no error)"=w495) -> ()  [unwired: 5 in, 2 out]
            n195 = call <vilib>:"Add State(s) to Queue__jki_lib_state_machine.vi"("State(s) in (\"\")"=w500) -> ("States Out"=w499:string)  [unwired: 14 in]
          }
          frame "---------- Log ----------" {
            # "All of these states should be handled by Handle Command, not here"
            n196 = Unbundle By Name(w501) -> ()  [unwired: 1 out]
            n197 = call <vilib>:"Add State(s) to Queue__jki_lib_state_machine.vi"("State(s) in (\"\")"=w505) -> ("States Out"=w504:string)  [unwired: 14 in]
          }
          frame "Log: Manager" {
            n198 = Unbundle By Name(w512) -> ("SelfRef"=w511:refnum<class "Instrument.Lockin.lvclass">)
            n199 = Unbundle By Name(w511) -> ("interval (ms)"=w509:u32, "DAQ State"=w508:T5, "mode"=w507:T2)
            n200 = case shown="\"Sweep\", Default" w506 {
              selector: w506 -> [_ w532]
              tunnel: [w522 w536] -> w510
              tunnel: w509 -> [_ w530]
              tunnel: w508 -> [w521 w535]
              tunnel: w507 -> [_ w534]
              frame "Sweep", Default {
                w517 = "UI: Update Status >> Log Sweep\nLog: Log Sweep" ("State(s) in Front (\"\")")
                n201 = Equal?(x=w521, y=Get_State-enum."sweeping") -> (x = y?=w525:bool)
                n202 = call <userlib>:"Periodic Trigger__ogtk.vi"("time (ms)"=u32 1000) -> ("Triggered"=w526:bool)  [unwired: 12 in, 2 out]
                n203 = Select(t="UI: Update Status >> Buffer Sweep\nData: Buffer" ("State(s) in Front (\"\")"), s=w525, f=w517) -> (s? t:f=w519:string)
                n204 = Select(t=w517, s=w526, f="") -> (s? t:f=w527:string)
                n205 = call <vilib>:"Add State(s) to Queue__jki_lib_state_machine.vi"("State(s) in Front (\"\")"=w519, "State(s) at Back (\"\")"=w527) -> ("States Out"=w522:string)  [unwired: 13 in]
              }
              frame "AO AI", "Results" {
                n206 = case shown="\"Results\", Default" w532 {
                  tunnel: ["UI: Update Status >> Log Results\nLog: Log Results" ("State(s) in Front (\"\")") "UI: Update Status >> Log AO\nLog: Log AO\nUI: Update Status >> Log AI\nLog: Log AI" ("State(s) in Front (\"\")")] -> w531
                  frame "Results", Default {
                  }
                  frame "AO AI" {
                  }
                }
                n207 = Equal?(x=w534, y=Lockin.Logging_Mode--Enum."enabled") -> (x = y?=w537:bool)
                n208 = Not Equal?(x=w535, y=Get_State-enum."sweeping") -> (x != y?=w538:bool)
                n209 = call <userlib>:"Periodic Trigger__ogtk.vi"("time (ms)"=w530) -> ("Triggered"=w529:bool)  [unwired: 12 in, 2 out]
                n210 = Compound Arithmetic op=AND(w529, w538, w537) -> (w528:bool)
                n211 = Select(t=w531, s=w528, f="" ("State(s) in Front (\"\")")) -> (s? t:f=w536:string)
              }
            }
            n212 = call <vilib>:"Add State(s) to Queue__jki_lib_state_machine.vi"("State(s) in Front (\"\")"=w510, "State(s) in (\"\")"=w516) -> ("States Out"=w515:string)  [unwired: 13 in]
          }
          frame "Log: Log AO" {
            n213 = Unbundle By Name(w546) -> ("SelfRef"=w543:refnum<class "Instrument.Lockin.lvclass">)
            n214 = call "Log AO.vi"("error in (no error)"=w544, "Instrument.Lockin in"=w543) -> ("error out"=w545:errorcluster)  [unwired: 8 in, 1 out]
            n215 = call <vilib>:"Add State(s) to Queue__jki_lib_state_machine.vi"("State(s) in (\"\")"=w549) -> ("States Out"=w548:string)  [unwired: 14 in]
          }
          frame "Log: Log AI" {
            n216 = Unbundle By Name(w553) -> ("SelfRef"=w551:refnum<class "Instrument.Lockin.lvclass">)
            n217 = call "Log AI.vi"("error in (no error)"=w550, "Instrument.Lockin in"=w551) -> ("error out"=w552:errorcluster)  [unwired: 8 in, 1 out]
            n218 = call <vilib>:"Add State(s) to Queue__jki_lib_state_machine.vi"("State(s) in (\"\")"=w556) -> ("States Out"=w555:string)  [unwired: 14 in]
          }
          frame "Log: Log Results" {
            n219 = Unbundle By Name(w560) -> ("SelfRef"=w559:refnum<class "Instrument.Lockin.lvclass">)
            n220 = call "Log Results.vi"("error in (no error)"=w558, "Instrument.Lockin in"=w559) -> ("error out"=w557:errorcluster)  [unwired: 8 in, 1 out]
            n221 = call <vilib>:"Add State(s) to Queue__jki_lib_state_machine.vi"("State(s) in (\"\")"=w563) -> ("States Out"=w562:string)  [unwired: 14 in]
          }
          frame "Log: Log Sweep" {
            n222 = Unbundle By Name(w565) -> ("SelfRef"=w570:refnum<class "Instrument.Lockin.lvclass">, "SweepWaveformsBuffer"=w567:T6)
            n223 = call "Log Sweep.vi"("error in (no error)"=w569, "SweepWaveforms"=w567, "Instrument.Lockin in"=w570) -> ("error out"=w568:errorcluster)  [unwired: 8 in]
            n224 = Bundle By Name(cluster=w565, "SweepWaveformsBuffer"=T6 {"AO_wfm"=[], "AI_wfm"=[], "X_wfm"=[], "Y_wfm"=[]}) -> (w566:T8)
            n225 = call <vilib>:"Add State(s) to Queue__jki_lib_state_machine.vi"("State(s) in (\"\")"=w573) -> ("States Out"=w572:string)  [unwired: 14 in]
          }
        }
      }
    }
    frame Error {
    }
  }
  n226 = call-parent "Process.vi"("error in"=w5, "Instrument"=w4) -> ("error out"=w2:errorcluster, "Instrument out"=→"Instrument.Lockin out":refnum<class "Instrument.Lockin.lvclass">)  [unwired: 8 in]
  n227 = Merge Errors(w2, w1) -> (→"error out":errorcluster)
